vi "Configure Accelerometer.vi"(5 "gyro range (deg/sec)":u16(ring)=250 items=["250"=250, "500"=500, "1000"=1000, "2000"=2000], 7 "accel range (g)":u16(ring)=2 items=["2"=2, "4"=4, "8"=8, "16"=16], 8 "error in (no error)":errorcluster, 11 "Accelerometer":T1) -> (0 "error out":errorcluster, 3 "Accelerometer out":T1)   [LabVIEW 2012]
doc: "Use this template to build a VI to use as a subVI."
uses:
  Accelerometer.ctl
  <vilib>/ni845x/ni845x.llb/ni845xControl.ctl
  <vilib>/ni845x/ni845x.llb/ni845xI2cConfiguration.ctl
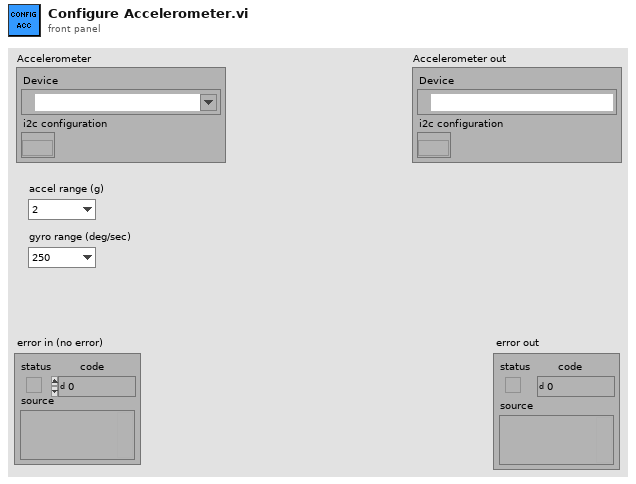
[diagram p1: front panel]
types:
  T1 = typedef "Accelerometer.ctl" = cluster{"Device":T2, "i2c configuration":T3}
  T2 = typedef "ni845xControl.ctl" = refnum<k21>
  T3 = typedef "ni845xI2cConfiguration.ctl" = refnum<k20>
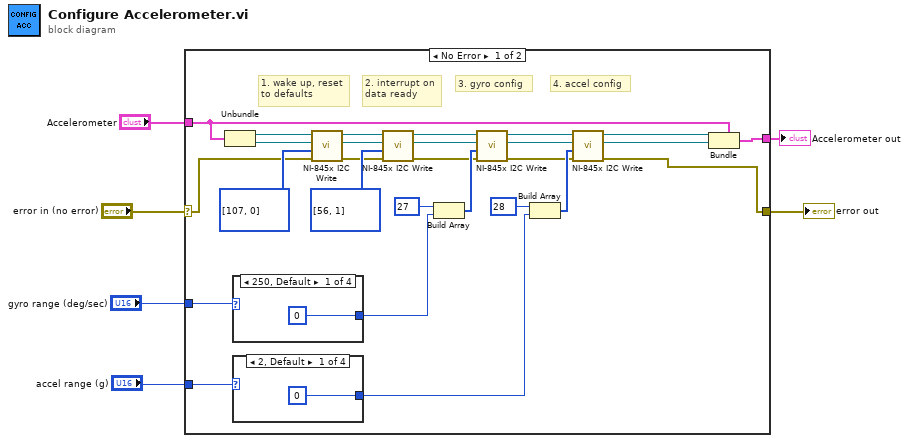
[diagram p0: block diagram]
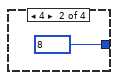
[diagram p2: hidden frame]
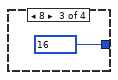
[diagram p3: hidden frame]
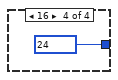
[diagram p4: hidden frame]
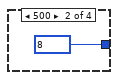
[diagram p5: hidden frame]
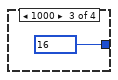
[diagram p6: hidden frame]
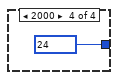
[diagram p7: hidden frame]
diagram:
  n1 = case shown="No Error" "error in (no error)" {
    selector: "error in (no error)" -> [w28 w43]
    tunnel: [w8 w43] -> w5
    tunnel: "Accelerometer" -> [w30 w42]
    tunnel: [w29 w42] -> w3
    tunnel: "gyro range (deg/sec)" -> [w23 _]
    tunnel: "accel range (g)" -> [w16 _]
    frame No Error {
      # "4. accel config"
      # "3. gyro config"
      # "2. interrupt on\ndata ready"
      # "1. wake up, reset\nto defaults"
      n2 = Unbundle(w30) -> ("Device"=w32:T2, "i2c configuration"=w31:T3)
      n3 = case shown="250, Default" w23 {
        tunnel: [u8 0 u8 8 u8 16 u8 24] -> w21
        frame 250, Default {
        }
        frame 500 {
        }
        frame 1000 {
        }
        frame 2000 {
        }
      }
      n4 = case shown="2, Default" w16 {
        tunnel: [u8 0 u8 8 u8 16 u8 24] -> w7
        frame 2, Default {
        }
        frame 4 {
        }
        frame 8 {
        }
        frame 16 {
        }
      }
      n5 = call <vilib>:"NI-845x I2C Write.vi"("error in (no error)"=w28, "write data"=u8[] [107, 0], "i2c configuration in"=w31, "device reference in"=w32) -> ("error out"=w24:errorcluster, "i2c configuration out"=w25:T3, "device reference out"=w26:T2)  [unwired: 5 in]
      n6 = call <vilib>:"NI-845x I2C Write.vi"("error in (no error)"=w24, "write data"=u8[] [56, 1], "i2c configuration in"=w25, "device reference in"=w26) -> ("error out"=w17:errorcluster, "i2c configuration out"=w18:T3, "device reference out"=w19:T2)  [unwired: 5 in]
      n7 = Build Array(u8 27, w21) -> (w20:u8[])
      n8 = call <vilib>:"NI-845x I2C Write.vi"("error in (no error)"=w17, "write data"=w20, "i2c configuration in"=w18, "device reference in"=w19) -> ("error out"=w11:errorcluster, "i2c configuration out"=w12:T3, "device reference out"=w13:T2)  [unwired: 5 in]
      n9 = Build Array(u8 28, w7) -> (w15:u8[])
      n10 = call <vilib>:"NI-845x I2C Write.vi"("error in (no error)"=w11, "write data"=w15, "i2c configuration in"=w12, "device reference in"=w13) -> ("error out"=w8:errorcluster, "i2c configuration out"=w9:T3, "device reference out"=w10:T2)  [unwired: 5 in]
      n11 = Bundle(cluster=w30, "Device"=w10, "i2c configuration"=w9) -> (w29:T1)
    }
    frame Error {
    }
  }
  "error out" <- w5
  "Accelerometer out" <- w3
